vi "Timer.vi"(8 "error in (no error)":errorcluster, 9 "Reset":bool, 10 "Pause":bool) -> (0 "error out":errorcluster, 1 "Elapsed?":bool, 2 "Elapsed TIme":dbl)   [LabVIEW 2013]
doc: "This subVI has following funcnality\n1.Pause- When it is pressed it stops the running elapsed time to the current value.\n2.Reset- Change the elapsed time value to zero.\n3.Elapsed; On- Time is elapsed\n Off- Time has not elapsed.\n4.Elapsed Time- Count the elapsed time"
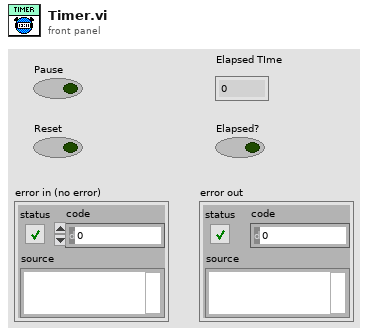
[diagram p1: front panel]
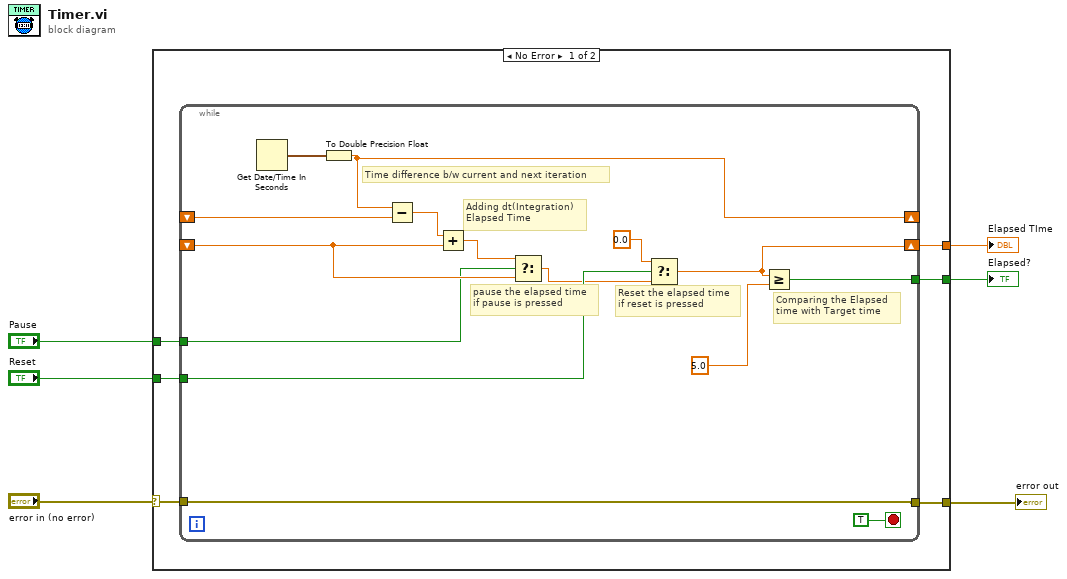
[diagram p0: block diagram]
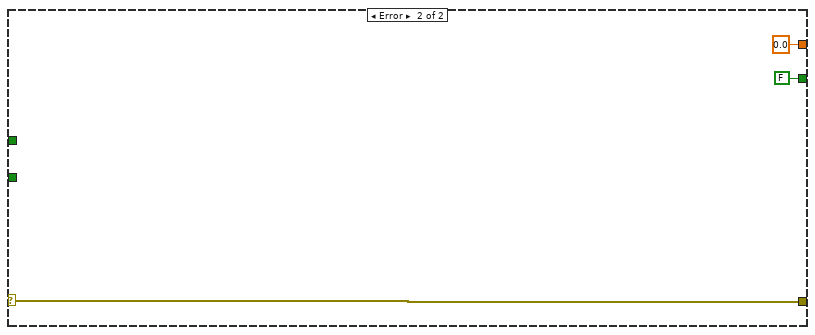
[diagram p2: hidden frame]
diagram:
  n1 = case shown="No Error" "error in (no error)" {
    selector: "error in (no error)" -> [w8 w30]
    tunnel: [w12 0.0 ("t")] -> w1
    tunnel: [w11 FALSE] -> w2
    tunnel: "Reset" -> [w10 _]
    tunnel: "Pause" -> [w9 _]
    tunnel: [w7 w30] -> w6
    frame No Error {
      n2 = while {
        shift-right: [w25] -> _
        shift-left: _ -> [w26]
        shift-right: [w22] -> w12
        shift-left: _ -> [w19]
        tunnel: [w15] -> w11
        tunnel: w10 -> [w23]
        tunnel: w9 -> [w17]
        tunnel: w8 -> [w16]
        tunnel: [w16] -> w7
        stop <- TRUE stop-if-true
        # "Comparing the Elapsed\ntime with Target time"
        # "Reset the elapsed time \nif reset is pressed"
        # "pause the elapsed time \nif pause is pressed"
        # "Adding dt(Integration)\nElapsed Time"
        # "Time difference b/w current and next iteration"
        n3 = Get Date/Time In Seconds() -> (seconds since 1Jan1904=w27:timestamp)
        n4 = To Double Precision Float(number=w27) -> (double precision float=w25:dbl)
        n5 = Subtract(x=w25, y=w26) -> (x-y=w24:dbl)
        n6 = Add(x=w24, y=w19) -> (x+y=w20:dbl)
        n7 = Select(t=w20, s=w17, f=w19) -> (s? t:f=w18:dbl)
        n8 = Select(t=0.0, s=w23, f=w18) -> (s? t:f=w22:dbl)
        n9 = Greater Or Equal?(x=w22, y=5.0) -> (x >= y?=w15:bool)
      }
    }
    frame Error {
    }
  }
  "error out" <- w6
  "Elapsed?" <- w2
  "Elapsed TIme" <- w1
